vi "Reset Control.vi"(0 "GEA2 Reference In":refnum<k24>, 11 "Error In":errorcluster) -> (4 "GEA2 Reference Out":refnum<k24>, 6 "Pass/Fail?":bool, 8 "Report Text":string, 15 "Error Out":errorcluster)   [LabVIEW 2016, in "TLMB.lvlib"]
doc: "Use this VI to reset the board."
uses:
  Projects/TLMB.lvlib
  Q:/Common/DLLs/GEA3/GeaCommunication.dll
  Common/DLLs/GEA3/GeaCommunication.dll
  Common/LabVIEW GEA2 Toolkit/LabVIEW_GEA2_Toolkit.lvlibp/type defs/ERD Write Data In.ctl
  Common/LabVIEW GEA2 Toolkit/LabVIEW_GEA2_Toolkit.lvlibp/type defs/Data Type.ctl
  Common/LabVIEW GEA2 Toolkit/LabVIEW_GEA2_Toolkit.lvlibp/type defs/Source_Destination.ctl
  Common/LabVIEW GEA2 Toolkit/LabVIEW_GEA2_Toolkit.lvlibp
panel:
  out "Time to fault code clear":dbl
  out "Time to fault code set (s)":dbl
  in  "Standalone?":bool
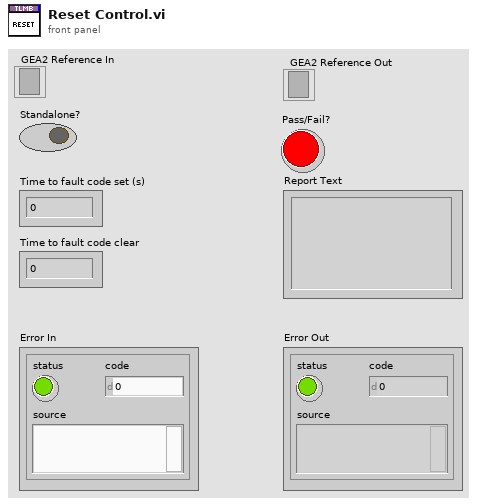
[diagram p1: front panel]
types:
  T1 = typedef "LabVIEW_GEA2_Toolkit.lvlibp/Source_Destination.ctl" = cluster{"Source":u8, "Destination":u8}
  T2 = typedef "LabVIEW_GEA2_Toolkit.lvlibp/ERD Write Data In.ctl" = cluster{"ERD Number":u16, "Data Type":T3, "Data":string}
  T3 = typedef "LabVIEW_GEA2_Toolkit.lvlibp/Data Type.ctl" = enum16{"string", "boolean", "uint8_t", "uint16_t", "uint32_t", "uint64_t", "int8_t", "int16_t", "int32_t", "int64_t"}
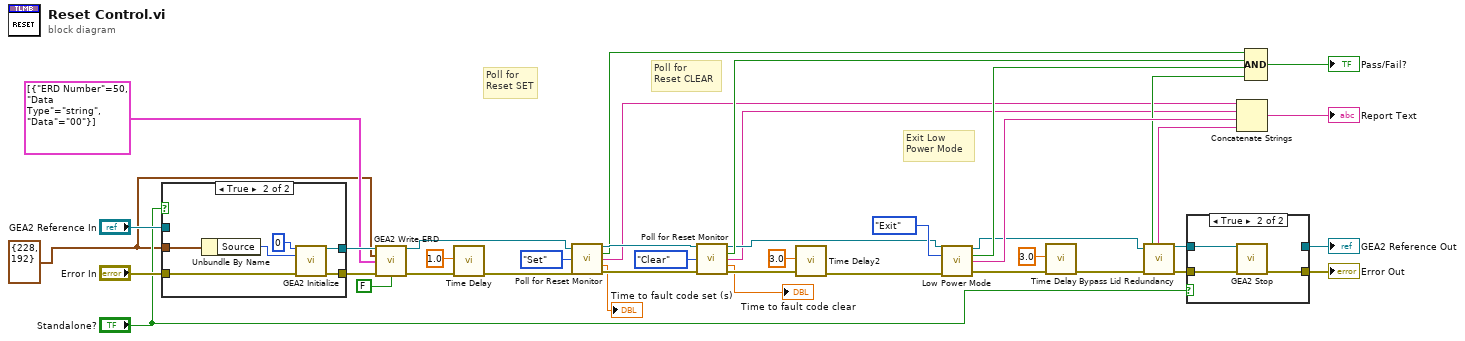
[diagram p0: block diagram]
diagram:
  w15 = T1 {"Source"=228, "Destination"=192} ("GEA Inputs")
  # "Exit Low \nPower Mode"
  # "Poll for\nReset CLEAR"
  # "Poll for\nReset SET"
  n1 = case shown="True" "Standalone?" {
    tunnel: "Error In" -> [w42 w49]
    tunnel: [w42 w48] -> w36
    tunnel: "GEA2 Reference In" -> [w43 _]
    tunnel: [w43 w47] -> w41
    tunnel: w15 -> [_ w45]
    frame False {
    }
    frame True {
      n2 = Unbundle By Name(w45) -> ("Source"=w46:u8)
      n3 = call "GEA2 Initialize.vi"("Board Index"=0, "Source Address"=w46, "error in"=w49) -> ("GEA2 Reference Out"=w47:refnum<k24>, "error out"=w48:errorcluster)  [unwired: 10 in, 1 out]
    }
  }
  n4 = call "GEA2 Write ERD.vi"("GEA2 Reference In"=w41, "GEA Inputs"=w15, "Write ERD List"=T2[] [{"ERD Number"=50, "Data Type"=enum."string", "Data"="00"}], "Error In"=w36, "Verify ERD Response?"=FALSE) -> ("GEA2 Reference Out"=w10:refnum<k24>, "Error Out"=w28:errorcluster)  [unwired: 8 in, 1 out]
  n5 = call "Time Delay"("error in (no error)"=w28, "Delay Time (s)"=1.0) -> ("error out"=w14:errorcluster)  [unwired: 9 in]
  n6 = call "Poll for Reset Monitor.vi"("GEA2 Reference In"=w10, "Status"=enum16{"Clear", "Set"}."Set", "Error In"=w14) -> ("GEA2 Reference Out"=w9:refnum<k24>, "Pass/Fail?"=w8:bool, "Report Text"=w3:string, "Time until condition met (s)"=→"Time to fault code set (s)":dbl, "Error Out"=w12:errorcluster)  [unwired: 8 in]
  n7 = call "Poll for Reset Monitor.vi"("GEA2 Reference In"=w9, "Status"=enum16{"Clear", "Set"}."Clear", "Error In"=w12) -> ("GEA2 Reference Out"=w6:refnum<k24>, "Pass/Fail?"=w7:bool, "Report Text"=w4:string, "Time until condition met (s)"=→"Time to fault code clear":dbl, "Error Out"=w5:errorcluster)  [unwired: 8 in]
  n8 = call "Time Delay2"("error in (no error)"=w5, "Delay Time (s)"=3.0) -> ("error out"=w22:errorcluster)  [unwired: 9 in]
  n9 = call "Low Power Mode.vi"("GEA2 Reference In"=w6, "Action"=enum16{"Enter", "Exit"}."Exit", "Error In"=w22) -> ("GEA2 Reference Out"=w18:refnum<k24>, "Pass/Fail?"=w30:bool, "Report Text"=w33:string, "Error Out"=w24:errorcluster)  [unwired: 9 in]
  n10 = call "Time Delay"("error in (no error)"=w24, "Delay Time (s)"=3.0) -> ("error out"=w21:errorcluster)  [unwired: 9 in]
  n11 = call "Bypass Lid Redundancy.vi"("GEA2 Reference In"=w18, "Error In"=w21) -> ("GEA2 Reference Out"=w19:refnum<k24>, "Pass/Fail?"=w17:bool, "Report Text"=w16:string, "Error Out"=w20:errorcluster)  [unwired: 10 in]
  n12 = case shown="True" "Standalone?" {
    tunnel: w20 -> [w51 w54]
    tunnel: [w51 w53] -> w40
    tunnel: [w50 _] -> w39
    tunnel: w19 -> [w50 w52]
    frame False {
    }
    frame True {
      n13 = call "GEA2 Stop.vi"("GEA2 Reference In"=w52, "Error In"=w54) -> ("Error Out"=w53:errorcluster)  [unwired: 13 in]
    }
  }
  "Error Out" <- w40
  "GEA2 Reference Out" <- w39
  n14 = Concatenate Strings(w3, w4, w33, w16) -> (→"Report Text":string)
  n15 = Compound Arithmetic op=AND(w8, w7, w30, w17) -> (→"Pass/Fail?":bool)
